vi "New Data.vi"(6 "dt":dbl, 8 "error in (no error)":errorcluster, 9 "t0":dbl, 10 "Data":dbl[][](array[numeric]), 11 "DataHandler in":refnum<class "DataHandler.lvclass">) -> (0 "error out":errorcluster, 3 "DataHandler out":refnum<class "DataHandler.lvclass">)   [LabVIEW 2020, in "VolatusData.lvlib" / "DataHandler.lvclass"]
uses:
  DataHandler.lvclass
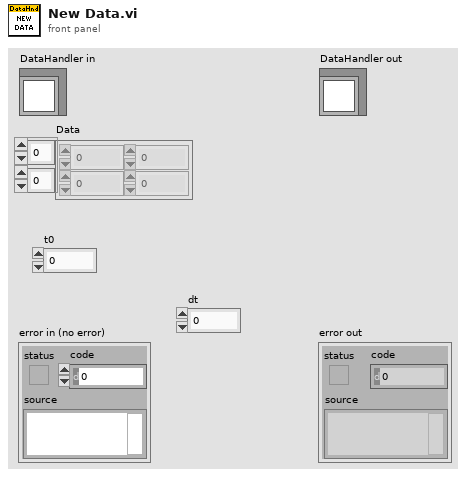
[diagram p1: front panel]
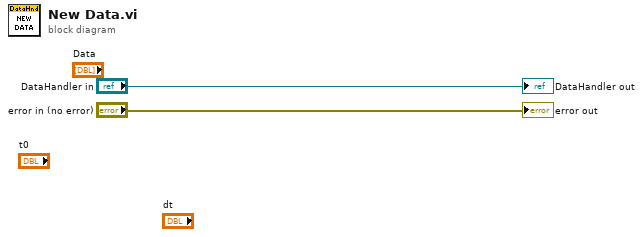
[diagram p0: block diagram]
diagram:
  "error out" <- "error in (no error)"
  "DataHandler out" <- "DataHandler in"
